vi "RMXWriteRead.vi"(8 "error in (no error)":errorcluster, 10 "Write Command/Query":string, 11 "VISA resource name":refnum<visa-resource-name>) -> (0 "error out":errorcluster, 2 "Response":string, 3 "VISA resource name out":refnum<visa-resource-name>)   [LabVIEW 2023]
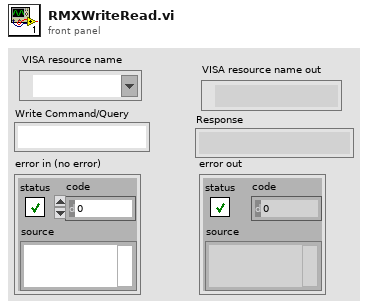
[diagram p1: front panel]
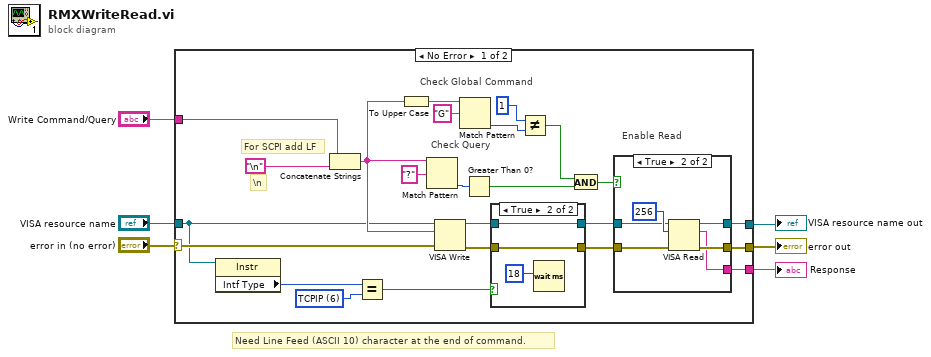
[diagram p0: block diagram]
diagram:
  # "Need Line Feed (ASCII 10) character at the end of command."
  n1 = case shown="No Error" "error in (no error)" {
    selector: "error in (no error)" -> [w16 w44]
    tunnel: "VISA resource name" -> [w10 w45]
    tunnel: [w14 w45] -> w3
    tunnel: [w15 w44] -> w5
    tunnel: "Write Command/Query" -> [w13 _]
    tunnel: [w12 _] -> w1
    frame No Error {
      w9 = u16 6 items=["GPIB"=1, "VXI"=2, "GPIB-VXI"=3, "Serial"=4, "PXI"=5, "TCPIP"=6, "USB"=7] ("Interface Information:Interface Type")
      # "\\n"
      # "For SCPI add LF"
      # "Check Global Command"
      # "Enable Read"
      # "Check Query"
      n2 = property class="Instr"(reference=w10) -> ("Intf Type"=w8:u16)  [unwired: 1 in, 2 out]
      n3 = Concatenate Strings(w13, "\n") -> (w11:string)
      n4 = Equal?(x=w8, y=w9) -> (x = y?=w7:bool)
      n5 = To Upper Case(1:w11) -> (0:w27:string)
      n6 = Match Pattern(string=w11, regular expression="?") -> (offset past match=w29:i32)  [unwired: 1 in, 3 out]
      n7 = VISA Write(VISA resource name=w10, write buffer=w11, error in (no error)=w16) -> (VISA resource name out=w21:refnum<visa-resource-name>, error out=w23:errorcluster)  [unwired: 1 out]
      n8 = Match Pattern(string=w27, regular expression="G") -> (offset past match=w26:i32)  [unwired: 1 in, 3 out]
      n9 = Greater Than 0?(x=w29) -> (x > 0?=w17:bool)
      n10 = case shown="True" w7 {
        tunnel: w23 -> [w31 w35]
        tunnel: [w31 w35] -> w22
        tunnel: w21 -> [w32 w34]
        tunnel: [w32 w34] -> w20
        frame False {
        }
        frame True {
          n11 = Wait (ms)(milliseconds to wait=u32 18) -> ()  [unwired: 1 out]
        }
      }
      n12 = Not Equal?(x=1, y=w26) -> (x != y?=w25:bool)
      n13 = And(x=w25, y=w17) -> (x .and. y?=w24:bool)
      n14 = case shown="True" w24 {
        tunnel: w22 -> [w36 w42]
        tunnel: w20 -> [w37 w41]
        tunnel: [w37 w40] -> w14
        tunnel: [w36 w39] -> w15
        tunnel: [_ w38] -> w12
        frame False {
        }
        frame True {
          n15 = VISA Read(VISA resource name=w41, byte count=u32 256 ("byte count (0)"), error in (no error)=w42) -> (VISA resource name out=w40:refnum<visa-resource-name>, read buffer=w38:string, error out=w39:errorcluster)  [unwired: 1 out]
        }
      }
    }
    frame Error {
    }
  }
  "VISA resource name out" <- w3
  "error out" <- w5
  "Response" <- w1
